vi "niDTS WLAN VHT Tx Test Set Parameters.vi"(0 "Dummy Test Handle in":T10, 7 "VHT Parameters":T1={"MCS Index"=0, "N Spatial Streams"=0, "Chains"=[TRUE, FALSE, FALSE, FALSE], "Bandwidth (Hz)"=enum."20 MHz", "Channel"=0, "Gard Interval"=enum."LONG", "FEC Coding"=enum."BCC", "Dut Tx Power (dBm)"=0.0, "16 symbols"=FALSE, "Payload Length (bytes)"=0, "Idle Interval (s)"=0.0, "External Attenuation (dB)"=[0.0, 0.0, 0.0, 0.0], "Acquisition "={"Acquisition Length Mode"=enum."AUTO", "Acquisition Length (s)"=0.0, "Auto Level"=FALSE}, "TXP Measurement"={"TXP Power Enable"=FALSE, "TXP Averages"=0}, "ModAcc Measurement"={"ModAcc Enable"=FALSE, "Header Detection"=enum."MANUAL", "Averages"=0, "CFO Estimation"=enum."PAMBLE", "Amplitude Tracking"=FALSE, "Channel Tracking"=FALSE, "Time Tracking"=FALSE, "Phase Tracking"=enum."NONE", "Clock Offset Est"=FALSE, "Impairments Est"=FALSE}, "SEM Measurement"={"SEM Enable"=FALSE, "SEM Averages"=0, "Auto Span Enable"=FALSE, "Frequency Span (Hz)"=0.0, "Measurement Type"=enum."Standard", "Mask Frequencies (Hz)"=[], "Mask Power Offsets (dB)"=[]}, "OBW Measurement"={"OBW Enable"=FALSE, "OBW Averages"=0}} {"Acquisition"."Acquisition Length (s)" format="%#_6p"; "SEM Measurement"."Frequency Span (Hz)" format="%#_6p"; "Idle Interval (s)" format="%_3p"}, 11 "error in (no error)":errorcluster) -> (4 "Dummy Test Handle out":T10, 15 "error out":errorcluster)   [LabVIEW 2014, in "niDTS WLAN.lvlib"]
uses:
  niDTS WLAN.lvlib
  Tx Test/Includes/niDTS WLAN Tx Test INC Handle.ctl
  Tx Test/Objects/BASE_class/niDTS WLAN Tx Test.lvclass
  Includes/niDTS WLAN VHT Tx Test INC Parameters.ctl
  Includes/niDTS WLAN INC CH BW.ctl
  Includes/niDTS WLAN INC GI.ctl
  Includes/niDTS WLAN INC FEC Coding.ctl
  Includes/niDTS WLAN DUT INC Acquisition Parameters.ctl
  Includes/niDTS WLAN INC TXP Measurement Parameters.ctl
  OFDM Tx Test/Includes/niDTS WLAN OFDM Tx Test INC ModAcc Measurement Parameters.ctl
  Includes/niDTS WLAN INC SEM Measurement Parameters.ctl
  Includes/niDTS WLAN INC OBW Measurement Parameters.ctl
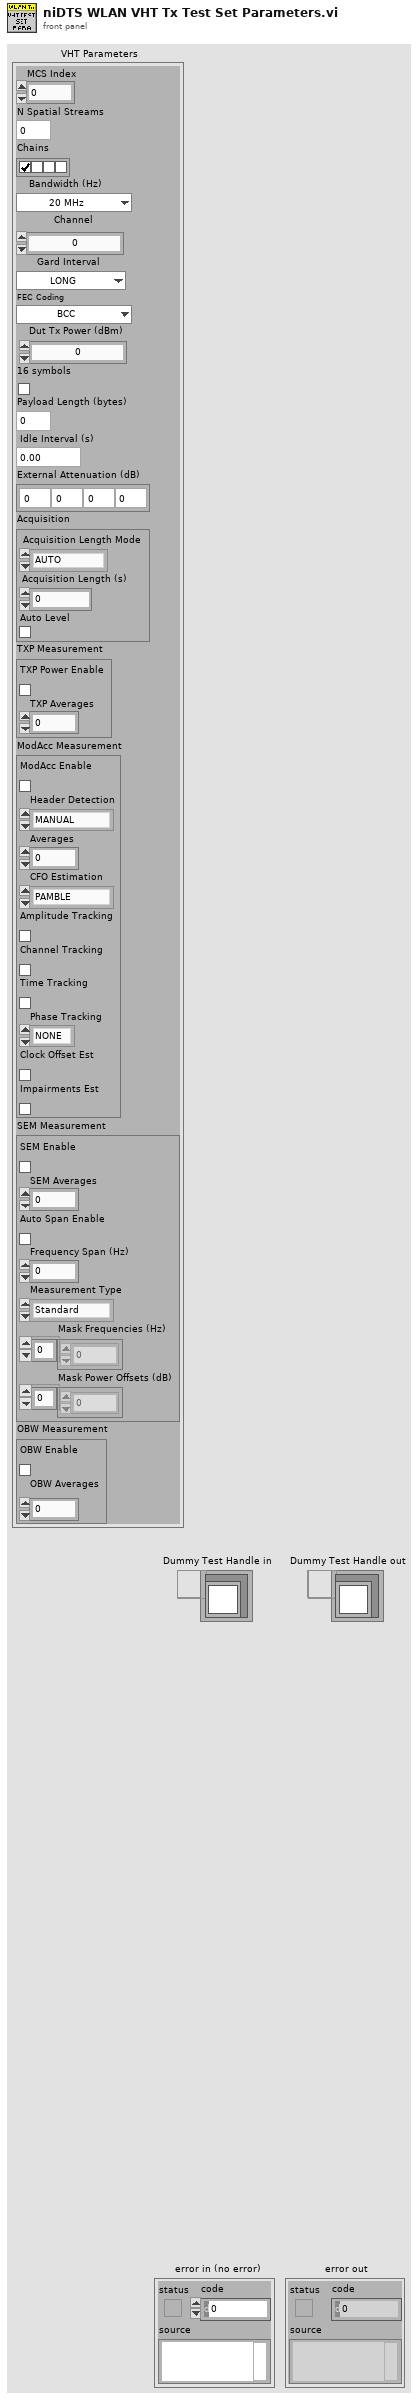
[diagram p1: front panel]
types:
  T1 = typedef "niDTS WLAN.lvlib/niDTS WLAN VHT Tx Test INC Parameters.ctl" = cluster{"MCS Index":i32, "N Spatial Streams":i32, "Chains":bool[], "Bandwidth (Hz)":T2, "Channel":i32, "Gard Interval":T3, "FEC Coding":T4, "Dut Tx Power (dBm)":dbl, "16 symbols":bool, "Payload Length (bytes)":i32, "Idle Interval (s)":dbl, "External Attenuation (dB)":dbl[], "Acquisition ":T5, "TXP Measurement":T6, "ModAcc Measurement":T7, "SEM Measurement":T8, "OBW Measurement":T9}
  T2 = typedef "niDTS WLAN.lvlib/niDTS WLAN INC CH BW.ctl" = enum16{"20 MHz", "40 MHz", "80 MHz", "160 MHz"}
  T3 = typedef "niDTS WLAN.lvlib/niDTS WLAN INC GI.ctl" = enum16{"LONG", "SHORT"}
  T4 = typedef "niDTS WLAN.lvlib/niDTS WLAN INC FEC Coding.ctl" = enum16{"BCC", "LDPC"}
  T5 = typedef "niDTS WLAN.lvlib/niDTS WLAN DUT INC Acquisition Parameters.ctl" = cluster{"Acquisition Length Mode":enum16{"AUTO", "MANUAL"}, "Acquisition Length (s)":dbl, "Auto Level":bool}
  T6 = typedef "niDTS WLAN.lvlib/niDTS WLAN INC TXP Measurement Parameters.ctl" = cluster{"TXP Power Enable":bool, "TXP Averages":i32}
  T7 = typedef "niDTS WLAN.lvlib/niDTS WLAN OFDM Tx Test INC ModAcc Measurement Parameters.ctl" = cluster{"ModAcc Enable":bool, "Header Detection":enum16{"MANUAL", "FIRST", "ALL"}, "Averages":i32, "CFO Estimation":enum16{"PAMBLE", "PDATA"}, "Amplitude Tracking":bool, "Channel Tracking":bool, "Time Tracking":bool, "Phase Tracking":enum16{"NONE", "STANDARD", "CSF", "INSTANT"}, "Clock Offset Est":bool, "Impairments Est":bool}
  T8 = typedef "niDTS WLAN.lvlib/niDTS WLAN INC SEM Measurement Parameters.ctl" = cluster{"SEM Enable":bool, "SEM Averages":i32, "Auto Span Enable":bool, "Frequency Span (Hz)":dbl, "Measurement Type":enum16{"Standard", "Legacy", "Custom"}, "Mask Frequencies (Hz)":dbl[], "Mask Power Offsets (dB)":dbl[]}
  T9 = typedef "niDTS WLAN.lvlib/niDTS WLAN INC OBW Measurement Parameters.ctl" = cluster{"OBW Enable":bool, "OBW Averages":i32}
  T10 = typedef "niDTS WLAN.lvlib/niDTS WLAN Tx Test INC Handle.ctl" = refnum<data-value>
  T11 = typedef "niDTS WLAN.lvlib/niDTS WLAN Tx Test INC Parameters.ctl" = cluster{"Standard":T12, "DSSS Data Rate (Mbps)":T13, "OFDM Data Rate (Mbps)":T14, "MCS Index":i32, "N spatial streams":i32, "Chains":bool[], "BandWidth (Hz)":T2, "Channel":i32, "Gard Interval":T3, "FEC Coding":T4, "Dut Tx Power":dbl, "16 symbols":bool, "payload length bytes":i32, "idle interval":dbl, "External Attenuation":dbl[], "Acquisition Parameters ":T5, "TXP Measurement Parameters":T6, "ModAcc Measurement Paramaters":T15, "ModAcc DSSS Paramaters":T16, "SEM Measurement Parameters":T8, "OBW Measurement Parameters":T9, "DSSS Power Ramp":T18, "Enable Traces":bool}
  T12 = typedef "niDTS WLAN.lvlib/niDTS WLAN INC Standard.ctl" = enum16{"802.11 b DSSS", "802.11 a/g OFDM", "802.11 n HT", "802.11 ac VHT"}
  T13 = typedef "niDTS WLAN.lvlib/niDTS WLAN INC DSSS Data Rate.ctl" = enum16{"1", "2", "5.5", "11"}
  T14 = typedef "niDTS WLAN.lvlib/niDTS WLAN INC OFDM Data Rate.ctl" = enum16{"6", "9", "12", "18", "24", "36", "48", "54"}
  T15 = typedef "niDTS WLAN.lvlib/niDTS WLAN INC ModAcc Measurement Parameters.ctl" = cluster{"ModAcc Enable":bool, "Header Detection":enum16{"MANUAL", "FIRST", "ALL"}, "Averages":i32, "Amplitude Tracking":bool, "Channel Tracking":bool, "Time Tracking":bool, "Phase Tracking":enum16{"NONE", "STANDARD", "CSF", "INSTANT"}, "Clock Offset Est":bool, "Impairments Est":bool, "CFO Estimation":enum16{"PAMBLE", "PDATA"}}
  T16 = typedef "niDTS WLAN.lvlib/niDTS WLAN INC DSSS ModAcc Measurement Parameters.ctl" = cluster{"DC Offset Compensation":bool, "Equalization":bool, "Phase Tracking":bool, "Chip Start Location":i16, "Max Chips Used":i16, "Pulse Shaping FilterType":T17, "Pulse Shaping Filter Coefficient":dbl}
  T17 = typedef "niDTS WLAN.lvlib/niDTS WLAN INC Pulse Shaping Filter Type.ctl" = enum16{"NONE", "RCOSINE", "RRCOSINE", "GAUSSIAN"}
  T18 = typedef "niDTS WLAN.lvlib/niDTS WLAN INC DSSS Power Ramp Parameters.ctl" = cluster{"Power Ramp Enable":bool, "Averages":i32, "Thresholds":cluster{"Up Low (%)":dbl, "Down Low (%)":dbl, "Up High (%)":dbl, "Down High (%)":dbl}}
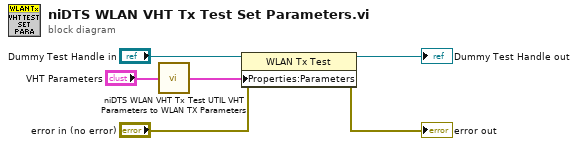
[diagram p0: block diagram]
diagram:
  n1 = call "niDTS WLAN VHT Tx Test UTIL VHT Parameters to WLAN TX Parameters.vi"("HT Parameters"="VHT Parameters") -> ("WLAN Tx Parameters"=w1:T11)  [unwired: 14 in]
  n2 = property class="WLAN Tx Test"(reference="Dummy Test Handle in", error in="error in (no error)", "Properties:Parameters"=w1) -> (reference out=→"Dummy Test Handle out":T10, error out=→"error out":errorcluster)
